vi "Store Configuration Parameters.vi"(8 "error in (no error)":errorcluster, 10 "refnum":T1, 11 "monitor configuration in":refnum<class "CCD monitor configuration.lvclass">) -> (0 "error out":errorcluster, 2 "refnum out":T1, 3 "monitor configuration out":refnum<class "CCD monitor configuration.lvclass">)   [LabVIEW 2016, in "CCD monitor.lvlib" / "CCD monitor configuration.lvclass"]
uses:
  <userlib>/Common Components/Hardware/Abstract System/Monitor/CCD monitor configuration.lvclass
  <vilib>/Utility/config.llb/Config Data RefNum.ctl
  <userlib>/Common Components/Hardware/CCD/CCD Configuration.lvclass
  <vilib>/Utility/config.llb/NI_LVConfig.lvlib
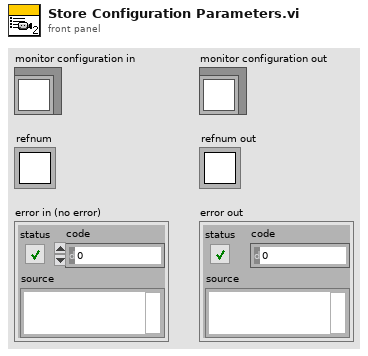
[diagram p1: front panel]
types:
  T1 = typedef "NI_LVConfig.lvlib/Config Data RefNum.ctl" = refnum<k1>
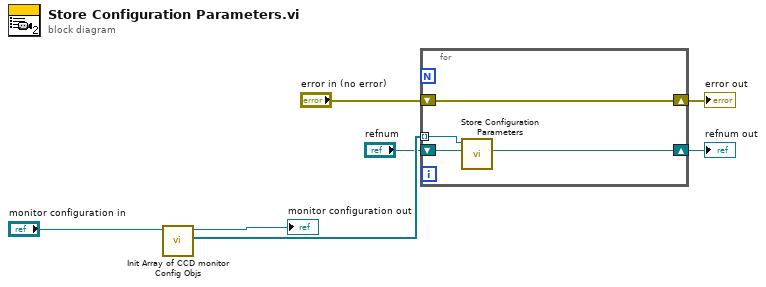
[diagram p0: block diagram]
diagram:
  n1 = call <userlib>:"Init Array of CCD monitor Config Objs.vi"("Hardware.lvlib:CCD monitor.lvlib:CCD monitor configuration.lvclass"="monitor configuration in") -> ("Array of CCD monitor"=w6:refnum<class "CCD Configuration.lvclass">[], "reference out"=→"monitor configuration out":refnum<class "CCD monitor configuration.lvclass">)  [unwired: 8 in, 1 out]
  n2 = for {
    tunnel: w6 -> [w11] mode=indexing
    shift-right: [w9] -> w3
    shift-left: "refnum" -> [w10]
    shift-right: [w8] -> w1
    shift-left: "error in (no error)" -> [w8]
    n3 = call-dynamic "Store Configuration Parameters.vi"("refnum"=w10, "CCD Configuration in"=w11) -> ("refnum out"=w9:T1)  [unwired: 7 in, 2 out]
  }
  "error out" <- w1
  "refnum out" <- w3
